vi "ADQUIRIR.vi"() -> ()   [LabVIEW 2021]
uses:
  <vilib>/MakerHub/LINX/Public/Peripherals/PWM/PWM Set Duty Cycle 1 Chan.vi
  <vilib>/MakerHub/LINX/Public/Peripherals/Analog/Analog Read 1 Chan.vi
  <vilib>/MakerHub/LINX/Public/Peripherals/Analog/Analog Read N Chans.vi
  <vilib>/MakerHub/LINX/Private/Local IO/LinxAnalogRead.vi
  <vilib>/MakerHub/LINX/Public/Utilities/Check Channel.vi
  <vilib>/MakerHub/LINX/Public/Utilities/Open Serial.vi
  <vilib>/MakerHub/LINX/Public/Peripherals/PWM/PWM Set Duty Cycle N Chans.vi
  <vilib>/MakerHub/LINX/Private/Utilties/Generate Error.vi
  <vilib>/MakerHub/LINX/LMH-LINX.lvlib
panel:
  in  "millisecond multiple":u32
  out "Waveform Chart":dynamicdata(graph)
  out "yk":dbl
  in  "uk":dbl
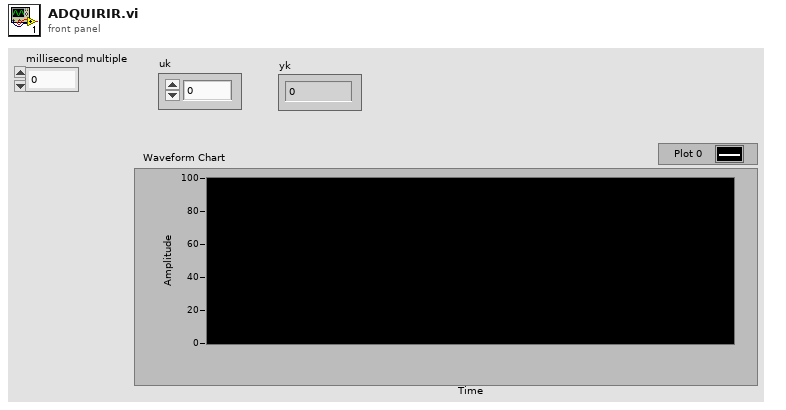
[diagram p1: front panel]
types:
  T1 = typedef "LMH-LINX.lvlib/LINX Ref.ctl" = cluster{"IO":T2, "Interface":T3, "LINX Device Config":T4}
  T2 = typedef "LMH-LINX.lvlib/Platform.ctl" = enum16{"Remote", "Local"}
  T3 = typedef "LMH-LINX.lvlib/Interface.ctl" = enum16{"Serial", "TCP"}
  T4 = typedef "LMH-LINX.lvlib/Device.lvlib/LINX Device Config.ctl" = cluster{"Interface":T3, "COM Port":refnum<visa-resource-name>, "TCP Configuration":T5, "Device Family":u8, "Device ID":u8, "Device Name":string, "TCP Ref":refnum<k5>, "Channels":T6}
  T5 = typedef "LMH-LINX.lvlib/Device.lvlib/TCP Config.ctl" = cluster{"IP Address":string, "Port":u16}
  T6 = typedef "LMH-LINX.lvlib/Channels.ctl" = cluster{"DI":u8[], "DO":u8[], "AI":u8[], "AO":u8[], "PWM":u8[], "QE":u8[], "UART":u8[], "I2C 2":u8[], "SPI":u8[], "CAN":u8[], "Servo":u8[], "AI Ref (V)":dbl, "AI Resolution (Bits)":u8, "AO Ref (V)":dbl, "AO Resolution (Bits)":u8}
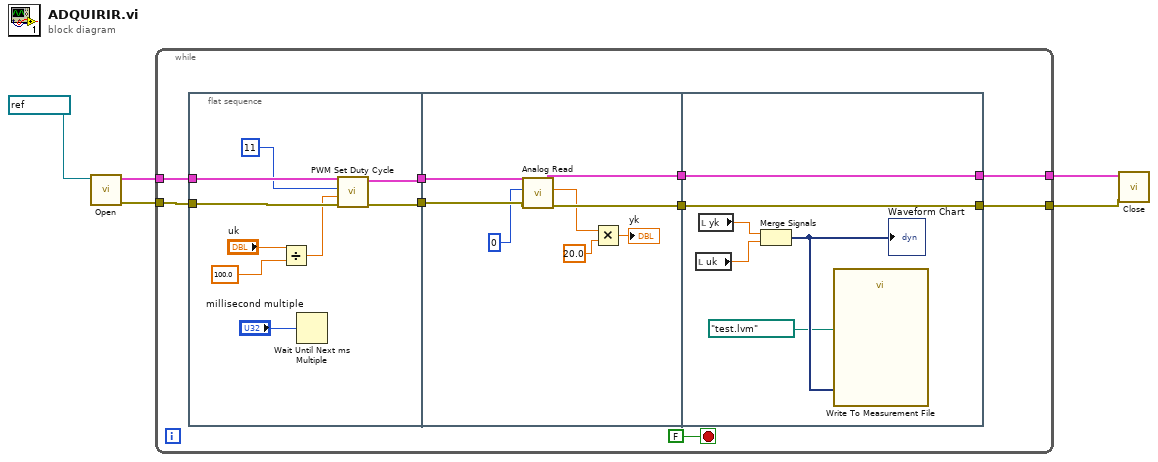
[diagram p0: block diagram]
diagram:
  n1 = call-poly <vilib>:"Open.vi"("Serial Port"=refnum<visa-resource-name> "COM3") -> ("Error Out"=w2:errorcluster, "LINX Resource"=w5:T1)  [unwired: 8 in, 1 out]
  n2 = while {
    tunnel: w5 -> [w14]
    tunnel: [w12] -> w4
    tunnel: w2 -> [w9]
    tunnel: [w7] -> w1
    stop <- FALSE stop-if-true
    n3 = flat-sequence {
      tunnel: w14 -> [w23]
      tunnel: [w21] -> w13
      tunnel: w9 -> [w22]
      tunnel: [w20] -> w8
      tunnel: w13 -> [w31]
      tunnel: [w30] -> w11
      tunnel: w8 -> [w29]
      tunnel: [w28] -> w6
      tunnel: [w37] -> w12
      tunnel: w11 -> [w37]
      tunnel: [w36] -> w7
      tunnel: w6 -> [w36]
      frame #0 {
        n4 = Divide(x="uk", y=100.0) -> (x/y=w16:dbl)
        n5 = Wait Until Next ms Multiple(millisecond multiple="millisecond multiple") -> ()  [unwired: 1 out]
        n6 = call-poly <vilib>:"PWM Set Duty Cycle.vi"("Error In"=w22, "Duty Cycle (0-1)"=w16, "PWM Channel"=u8 11, "LINX Resource"=w23) -> ("Error Out"=w20:errorcluster, "LINX Resource"=w21:T1)  [unwired: 6 in]
      }
      frame #1 {
        n7 = call-poly <vilib>:"Analog Read.vi"("Error In"=w29, "Analog Channel"=u8 0, "LINX Resource"=w31) -> ("Error Out"=w28:errorcluster, "Voltage"=w26:dbl, "LINX Resource"=w30:T1)  [unwired: 5 in, 1 out]
        n8 = Multiply(x=w26, y=20.0) -> (x*y=→"yk":dbl)
      }
      frame #2 {
        n9 = local read "uk"() -> (w34:dbl)
        n10 = local read "yk"() -> (w35:dbl)
        n11 = Merge Signals(w35, w34) -> (w33:dynamicdata)
        "Waveform Chart" <- w33
        n12 = call "Write To Measurement File"("Signals"=w33, "Filename"=path "test.lvm") -> ()  [unwired: 15 in, 3 out]
      }
    }
  }
  n13 = call <vilib>:"Close.vi"("Error In"=w1, "LINX Resource"=w4) -> ()  [unwired: 9 in, 1 out]
